vi "HS_AppendConsole.vi"(4 "Show Reply Binary?":bool=TRUE, 6 "Show Send Binary?":bool=TRUE, 8 "Reply":string, 9 "Console in":string, 10 "Send":string, 11 "Command":string="ENABLE FB:\nSend: %s\nReply: %s") -> (1 "Console Out":string)   [LabVIEW 2016]
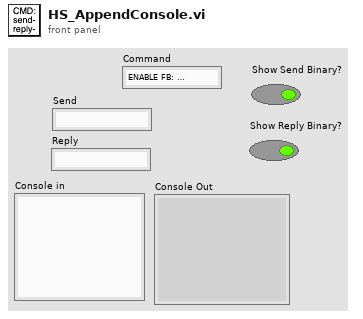
[diagram p1: front panel]
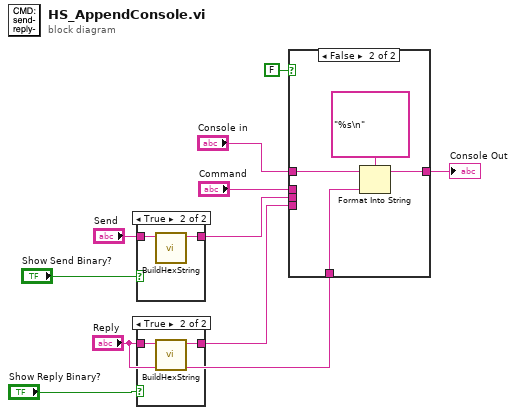
[diagram p0: block diagram]
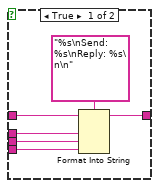
[diagram p2: hidden frame]
diagram:
  n1 = case shown="True" "Show Send Binary?" {
    tunnel: [w11 w13] -> w10
    tunnel: "Send" -> [w11 w12]
    frame False {
    }
    frame True {
      n2 = call <userlib>:"BuildHexString.vi"("Binary"=w12) -> ("String"=w13:string)  [unwired: 10 in]
    }
  }
  n3 = case shown="True" "Show Reply Binary?" {
    tunnel: [w14 w16] -> w3
    tunnel: "Reply" -> [w14 w15]
    frame False {
    }
    frame True {
      n4 = call <userlib>:"BuildHexString.vi"("Binary"=w15) -> ("String"=w16:string)  [unwired: 10 in]
    }
  }
  n5 = case shown="False" FALSE {
    tunnel: w10 -> [w22 _]
    tunnel: [w21 w26] -> w8
    tunnel: "Command" -> [w20 _]
    tunnel: "Console in" -> [w18 w24]
    tunnel: w3 -> [w17 _]
    tunnel: "Reply" -> [_ w23]
    frame True {
      n6 = Format Into String(format string="%s\nSend: %s\nReply: %s\n\n", initial string=w18, w20, w22, w17) -> (resulting string=w21:string)  [unwired: 1 in, 1 out]
    }
    frame False {
      n7 = Format Into String(format string="%s\n", initial string=w24, w23) -> (resulting string=w26:string)  [unwired: 1 in, 1 out]
    }
  }
  "Console Out" <- w8
